vi "string parse mathematica list assosiated array.vi"(6 "pattern":string="[\\\\\\s\\n]*(\\d+)[\\\\\\s\\n]*\\-\\>[\\\\\\s\\n]*\\<\\|((.|\\n)+?)\\|\\>[\\\\\\s\\n]*\\,", 7 "derivative":T2=enum."parse string", 8 "array of inds":dbl[](array[numeric]), 10 "Map IN":map{i32, map{T1, dbl}}(c390), 11 "string IN":string="\n8048 -> <|\"\\[Zeta]\" -> 0.264284777894, \"\\[Tau]1\" -> 0.029921918685, \n   \"\\[Tau]S\" -> 0.192386764745, \"\\[Tau]N\" -> 0.181403587913, \n   \"\\[Tau]C\" -> 0.001052808010, \"\\[Kappa]0\" -> 0.000000000660, \n   \"mm1\" -> 0.000000000000, \"mm2\" -> 0.000000000000, \n   \"mm3\" -> 0.000000000000, \"T\" -> 0.170000000000, \n   \"B\" -> 12, \"\\[Theta]\" -> 0.000000000000|>, \n8049 -> <|\"\\[Zeta]\" -> 0.201102232421, \"\\[Tau]1\" -> 0.027404257658, \n   \"\\[Tau]S\" -> 0.119081991530, \"\\[Tau]N\" -> 0.102233037825, \n   \"\\[Tau]C\" -> 0.001034759526, \"\\[Kappa]0\" -> 0.000000000924, \n   \"mm1\" -> 0.000000000000, \"mm2\" -> 0.000000000000, \n   \"mm3\" -> 0.000000000000, \"T\" -> 0.200000000000, \n   \"B\" -> 12, \"\\[Theta]\" -> 0.000000000000|>, \n8050 -> <|\"\\[Zeta]\" -> 0.169063131197, \"\\[Tau]1\" -> 0.023551252455, \n   \"\\[Tau]S\" -> 0.088556796938, \"\\[Tau]N\" -> 0.073591360902, \n   \"\\[Tau]C\" -> 0.001008773464, \"\\[Kappa]0\" -> 0.000000001052, \n   \"mm1\" -> 0.000000000000, \"mm2\" -> 0.000000000000, \n   \"mm3\" -> 0.000000000000, \"T\" -> 0.220000000000, \n   \"B\" -> 12, \"\\[Theta]\" -> 0.000000000000|>, \n8051 -> <|\"\\[Zeta]\" -> 0.091539753140, \"\\[Tau]1\" -> 0.021589342173, \n   \"\\[Tau]S\" -> 0.069591266812, \"\\[Tau]N\" -> 0.024713101747, \n   \"\\[Tau]C\" -> 0.001578835918, \"\\[Kappa]0\" -> 0.000000001376, \n   \"mm1\" -> 0.000000000000, \"mm2\" -> 0.000000000000, \n   \"mm3\" -> 0.000000000000, \"T\" -> 0.280000000000, \n   \"B\" -> 12, \"\\[Theta]\" -> 0.000000000000|>, \n8052 -> <|\"\\[Zeta]\" -> 0.064241434685, \"\\[Tau]1\" -> 0.021883189624, \n   \"\\[Tau]S\" -> 0.054526069267, \"\\[Tau]N\" -> 0.012051949674, \n   \"\\[Tau]C\" -> 0.001858120134, \"\\[Kappa]0\" -> 0.000000001749, \n   \"mm1\" -> 0.000000000000, \"mm2\" -> 0.000000000000, \n   \"mm3\" -> 0.000000000000, \"T\" -> 0.330000000000, \n   \"B\" -> 12, \"\\[Theta]\" -> 0.000000000000|>, \n8053 -> <|\"\\[Zeta]\" -> 0.046671238462, \"\\[Tau]1\" -> 0.021035137247, \n   \"\\[Tau]S\" -> 0.044251032051, \"\\[Tau]N\" -> 0.006393660877, \n   \"\\[Tau]C\" -> 0.002341606240, \"\\[Kappa]0\" -> 0.000000002165, \n   \"mm1\" -> 0.000000000000, \"mm2\" -> 0.000000000000, \n   \"mm3\" -> 0.000000000000, \"T\" -> 0.400000000000, \n   \"B\" -> 12, \"\\[Theta]\" -> 0.000000000000|>, \n 8054 -> <|\"\\[Zeta]\" -> 0.036507468942, \"\\[Tau]1\" -> 0.016809078537, \n   \"\\[Tau]S\" -> 0.036180977899, \"\\[Tau]N\" -> 0.004191377428, \n   \"\\[Tau]C\" -> 0.002304673955, \"\\[Kappa]0\" -> 0.000000002675, \n   \"mm1\" -> 0.000000000000, \"mm2\" -> 0.000000000000, \n   \"mm3\" -> 0.000000000000, \"T\" -> 0.480000000000, \n   \"B\" -> 12, \"\\[Theta]\" -> 0.000000000000|>, \n 8055 -> <|\"\\[Zeta]\" -> 0.030833243094, \"\\[Tau]1\" -> 0.018820733306, \n   \"\\[Tau]S\" -> 0.030309186701, \"\\[Tau]N\" -> 0.002241639015, \n   \"\\[Tau]C\" -> 0.002272740822, \"\\[Kappa]0\" -> 0.000000003352, \n   \"mm1\" -> 0.000000000000, \"mm2\" -> 0.000000000000, \n   \"mm3\" -> 0.000000000000, \"T\" -> 0.580000000000, \n   \"B\" -> 12, \"\\[Theta]\" -> 0.000000000000|>, \n 8056 -> <|\"\\[Zeta]\" -> 0.019920170845, \"\\[Tau]1\" -> 0.016368892412, \n   \"\\[Tau]S\" -> 0.030579536580, \"\\[Tau]N\" -> 0.001736017565, \n   \"\\[Tau]C\" -> 0.004971418152, \"\\[Kappa]0\" -> 0.000000004410, \n   \"mm1\" -> 0.000000000000, \"mm2\" -> 0.000000000000, \n   \"mm3\" -> 0.000000000000, \"T\" -> 0.680000000000, \n   \"B\" -> 12, \"\\[Theta]\" -> 0.000000000000|>, \n 8057 -> <|\"\\[Zeta]\" -> 0.017558473054, \"\\[Tau]1\" -> 0.014545104284, \n   \"\\[Tau]S\" -> 0.022979681288, \"\\[Tau]N\" -> 0.000840829385, \n   \"\\[Tau]C\" -> 0.005228030240, \"\\[Kappa]0\" -> 0.000000006068, \n   \"mm1\" -> 0.000000000000, \"mm2\" -> 0.000000000000, \n   \"mm3\" -> 0.000000000000, \"T\" -> 0.910000000000, \n   \"B\" -> 12, \"\\[Theta]\" -> 0.000000000000|>, \n 8058 -> <|\"\\[Zeta]\" -> 0.011916480594, \"\\[Tau]1\" -> 0.012551282481, \n   \"\\[Tau]S\" -> 0.018233218660, \"\\[Tau]N\" -> 0.000345702746, \n   \"\\[Tau]C\" -> 0.004699451527, \"\\[Kappa]0\" -> 0.000000008451, \n   \"mm1\" -> 0.000000000000, \"mm2\" -> 0.000000000000, \n   \"mm3\" -> 0.000000000000, \"T\" -> 1.230000000000, \n   \"B\" -> 12, \"\\[Theta]\" -> 0.000000000000|>, \n 8059 -> <|\"\\[Zeta]\" -> 0.012831327568, \"\\[Tau]1\" -> 0.013315909415, \n   \"\\[Tau]S\" -> 0.012590836847, \"\\[Tau]N\" -> 0.000065003013, \n   \"\\[Tau]C\" -> 0.005276356243, \"\\[Kappa]0\" -> 0.000000013610, \n   \"mm1\" -> 0.000000000000, \"mm2\" -> 0.000000000000, \n   \"mm3\" -> 0.000000000000, \"T\" -> 1.970000000000, \n   \"B\" -> 12, \"\\[Theta]\" -> 0.000000000000|>, \n 8060 -> <|\"\\[Zeta]\" -> 0.019774146838, \"\\[Tau]1\" -> 0.013257273421, \n   \"\\[Tau]S\" -> 0.007064131508, \"\\[Tau]N\" -> 0.000028000819, \n   \"\\[Tau]C\" -> 0.006942241845, \"\\[Kappa]0\" -> 0.000000023477, \n   \"mm1\" -> 0.000000000000, \"mm2\" -> 0.000000000000, \n   \"mm3\" -> 0.000000000000, \"T\" -> 3.190000000000, \n   \"B\" -> 12, \"\\[Theta]\" -> 0.000000000000|>, \n 8061 -> <|\"\\[Zeta]\" -> 0.029251354442, \"\\[Tau]1\" -> 0.014634751206, \n   \"\\[Tau]S\" -> 0.003873958746, \"\\[Tau]N\" -> 0.000007000487, \n   \"\\[Tau]C\" -> 0.006827504775, \"\\[Kappa]0\" -> 0.000000056438, \n   \"mm1\" -> 0.000000000000, \"mm2\" -> 0.000000000000, \n   \"mm3\" -> 0.000000000000, \"T\" -> 5.820000000000, \n   \"B\" -> 12, \"\\[Theta]\" -> 0.000000000000 |>, \n   \n 8070 -> <|\"\\[Zeta]\" -> 0.192260325342, \"\\[Tau]1\" -> 0.068971960572, \n   \"\\[Tau]S\" -> 0.034724103146, \"\\[Tau]N\" -> 0.116916926394, \n   \"\\[Tau]C\" -> 0.001339007531, \"\\[Kappa]0\" -> 0.000000000920, \n   \"mm1\" -> 0.000000000000, \"mm2\" -> 0.000000000000, \n   \"mm3\" -> 0.000000000000, \"T\" -> 0.200000000000, \n   \"B\" -> 12, \"\\[Theta]\" -> 90.000000000000 |>, \n   \n 8071 -> <|\"\\[Zeta]\" -> 0.287121975239, \"\\[Tau]1\" -> 0.116231019165, \n   \"\\[Tau]S\" -> 0.066964365948, \"\\[Tau]N\" -> 1.031943818405, \n   \"\\[Tau]C\" -> 0.001579683432, \"\\[Kappa]0\" -> 0.000000000546, \n   \"mm1\" -> 0.000000000000, \"mm2\" -> 0.000000000000, \n   \"mm3\" -> 0.000000000000, \"T\" -> 0.140000000000, \n   \"B\" -> 12, \"\\[Theta]\" -> 90.000000000000 |>, \n   \n 8072 -> <|\"\\[Zeta]\" -> 0.256563977847, \"\\[Tau]1\" -> 0.091128230148, \n   \"\\[Tau]S\" -> 0.042349271948, \"\\[Tau]N\" -> 0.264223732455, \n   \"\\[Tau]C\" -> 0.001175524600, \"\\[Kappa]0\" -> 0.000000000659, \n   \"mm1\" -> 0.000000000000, \"mm2\" -> 0.000000000000, \n   \"mm3\" -> 0.000000000000, \"T\" -> 0.180000000000, \n   \"B\" -> 12, \"\\[Theta]\" -> 90.000000000000|>, \n 8073 -> <|\"\\[Zeta]\" -> 0.166463706425, \"\\[Tau]1\" -> 0.068258677765, \n   \"\\[Tau]S\" -> 0.032169678694, \"\\[Tau]N\" -> 0.089325850968, \n   \"\\[Tau]C\" -> 0.001296501731, \"\\[Kappa]0\" -> 0.000000001072, \n   \"mm1\" -> 0.000000000000, \"mm2\" -> 0.000000000000, \n   \"mm3\" -> 0.000000000000, \"T\" -> 0.220000000000, \n   \"B\" -> 12, \"\\[Theta]\" -> 90.000000000000|>, \n 8074 -> <|\"\\[Zeta]\" -> 0.096966986681, \"\\[Tau]1\" -> 0.051268159149, \n   \"\\[Tau]S\" -> 0.027100433808, \"\\[Tau]N\" -> 0.035158364681, \n   \"\\[Tau]C\" -> 0.001794012368, \"\\[Kappa]0\" -> 0.000000001377, \n   \"mm1\" -> 0.000000000000, \"mm2\" -> 0.000000000000, \n   \"mm3\" -> 0.000000000000, \"T\" -> 0.270000000000, \n   \"B\" -> 12, \"\\[Theta]\" -> 90.000000000000|>, \n 8075 -> <|\"\\[Zeta]\" -> 0.069751073871, \"\\[Tau]1\" -> 0.043839592936, \n   \"\\[Tau]S\" -> 0.023745040482, \"\\[Tau]N\" -> 0.017573258627, \n   \"\\[Tau]C\" -> 0.001911807541, \"\\[Kappa]0\" -> 0.000000001743, \n   \"mm1\" -> 0.000000000000, \"mm2\" -> 0.000000000000, \n   \"mm3\" -> 0.000000000000, \"T\" -> 0.330000000000, \n   \"B\" -> 12, \"\\[Theta]\" -> 90.000000000000|>, \n 8076 -> <|\"\\[Zeta]\" -> 0.051456166730, \"\\[Tau]1\" -> 0.036962114127, \n   \"\\[Tau]S\" -> 0.021589166615, \"\\[Tau]N\" -> 0.010172333923, \n   \"\\[Tau]C\" -> 0.002367575609, \"\\[Kappa]0\" -> 0.000000002122, \n   \"mm1\" -> 0.000000000000, \"mm2\" -> 0.000000000000, \n   \"mm3\" -> 0.000000000000, \"T\" -> 0.390000000000, \n   \"B\" -> 12, \"\\[Theta]\" -> 90.000000000000|>, \n 8077 -> <|\"\\[Zeta]\" -> 0.038526442831, \"\\[Tau]1\" -> 0.026952038906, \n   \"\\[Tau]S\" -> 0.019853633024, \"\\[Tau]N\" -> 0.005229312619, \n   \"\\[Tau]C\" -> 0.002387050238, \"\\[Kappa]0\" -> 0.000000002669, \n   \"mm1\" -> 0.000000000000, \"mm2\" -> 0.000000000000, \n   \"mm3\" -> 0.000000000000, \"T\" -> 0.480000000000, \n   \"B\" -> 12, \"\\[Theta]\" -> 90.000000000000|>, \n 8078 -> <|\"\\[Zeta]\" -> 0.031217986851, \"\\[Tau]1\" -> 0.022324330444, \n   \"\\[Tau]S\" -> 0.018861062526, \"\\[Tau]N\" -> 0.002718571339, \n   \"\\[Tau]C\" -> 0.002455004531, \"\\[Kappa]0\" -> 0.000000003343, \n   \"mm1\" -> 0.000000000000, \"mm2\" -> 0.000000000000, \n   \"mm3\" -> 0.000000000000, \"T\" -> 0.580000000000, \n   \"B\" -> 12, \"\\[Theta]\" -> 90.000000000000|>, \n 8079 -> <|\"\\[Zeta]\" -> 0.020568815513, \"\\[Tau]1\" -> 0.023045965648, \n   \"\\[Tau]S\" -> 0.020791387386, \"\\[Tau]N\" -> 0.002229171297, \n   \"\\[Tau]C\" -> 0.004427475438, \"\\[Kappa]0\" -> 0.000000004398, \n   \"mm1\" -> 0.000000000000, \"mm2\" -> 0.000000000000, \n   \"mm3\" -> 0.000000000000, \"T\" -> 0.680000000000, \n   \"B\" -> 12, \"\\[Theta]\" -> 90.000000000000|>, \n 8080 -> <|\"\\[Zeta]\" -> 0.016159836955, \"\\[Tau]1\" -> 0.019958638777, \n   \"\\[Tau]S\" -> 0.018730096307, \"\\[Tau]N\" -> 0.000899236968, \n   \"\\[Tau]C\" -> 0.005152267403, \"\\[Kappa]0\" -> 0.000000006087, \n   \"mm1\" -> 0.000000000000, \"mm2\" -> 0.000000000000, \n   \"mm3\" -> 0.000000000000, \"T\" -> 0.910000000000, \n   \"B\" -> 12, \"\\[Theta]\" -> 90.000000000000|>, \n 8081 -> <|\"\\[Zeta]\" -> 0.014495870556, \"\\[Tau]1\" -> 0.019990087457, \n   \"\\[Tau]S\" -> 0.016832201384, \"\\[Tau]N\" -> 0.000455517238, \n   \"\\[Tau]C\" -> 0.005555782498, \"\\[Kappa]0\" -> 0.000000008420, \n   \"mm1\" -> 0.000000000000, \"mm2\" -> 0.000000000000, \n   \"mm3\" -> 0.000000000000, \"T\" -> 1.230000000000, \n   \"B\" -> 12, \"\\[Theta]\" -> 90.000000000000|>, \n 8082 -> <|\"\\[Zeta]\" -> 0.014043763709, \"\\[Tau]1\" -> 0.018292068543, \n   \"\\[Tau]S\" -> 0.011311396743, \"\\[Tau]N\" -> 0.000128802259, \n   \"\\[Tau]C\" -> 0.008087849636, \"\\[Kappa]0\" -> 0.000000014258, \n   \"mm1\" -> 0.000000000000, \"mm2\" -> 0.000000000000, \n   \"mm3\" -> 0.000000000000, \"T\" -> 2.050000000000, \n   \"B\" -> 12, \"\\[Theta]\" -> 90.000000000000|>, \n 8083 -> <|\"\\[Zeta]\" -> 0.016187684631, \"\\[Tau]1\" -> 0.018325345271, \n   \"\\[Tau]S\" -> 0.007510087776, \"\\[Tau]N\" -> 0.000028419157, \n   \"\\[Tau]C\" -> 0.008115463080, \"\\[Kappa]0\" -> 0.000000024747, \n   \"mm1\" -> 0.000000000000, \"mm2\" -> 0.000000000000, \n   \"mm3\" -> 0.000000000000, \"T\" -> 3.310000000000, \n   \"B\" -> 12, \"\\[Theta]\" -> 90.000000000000|>, \n 8084 -> <|\"\\[Zeta]\" -> 0.027897403691, \"\\[Tau]1\" -> 0.014639690770, \n   \"\\[Tau]S\" -> 0.004105291179, \"\\[Tau]N\" -> 0.000006999171, \n   \"\\[Tau]C\" -> 0.007414449545, \"\\[Kappa]0\" -> 0.000000059701, \n   \"mm1\" -> 0.000000000000, \"mm2\" -> 0.000000000000, \n   \"mm3\" -> 0.000000000000, \"T\" -> 6.000000000000, \n   \"B\" -> 12, \"\\[Theta]\" -> 90.000000000000|>,") -> (2 "Map OUT":map{i32, map{T1, dbl}}(c390), 3 "string out":string="\n8048 -> <|\"\\[Zeta]\" -> 0.264284777894, \"\\[Tau]1\" -> 0.029921918685, \n   \"\\[Tau]S\" -> 0.192386764745, \"\\[Tau]N\" -> 0.181403587913, \n   \"\\[Tau]C\" -> 0.001052808010, \"\\[Kappa]0\" -> 0.000000000660, \n   \"mm1\" -> 0.000000000000, \"mm2\" -> 0.000000000000, \n   \"mm3\" -> 0.000000000000, \"T\" -> 0.170000000000, \n   \"B\" -> 12, \"\\[Theta]\" -> 0.000000000000|>, \n8049 -> <|\"\\[Zeta]\" -> 0.201102232421, \"\\[Tau]1\" -> 0.027404257658, \n   \"\\[Tau]S\" -> 0.119081991530, \"\\[Tau]N\" -> 0.102233037825, \n   \"\\[Tau]C\" -> 0.001034759526, \"\\[Kappa]0\" -> 0.000000000924, \n   \"mm1\" -> 0.000000000000, \"mm2\" -> 0.000000000000, \n   \"mm3\" -> 0.000000000000, \"T\" -> 0.200000000000, \n   \"B\" -> 12, \"\\[Theta]\" -> 0.000000000000|>, \n8050 -> <|\"\\[Zeta]\" -> 0.169063131197, \"\\[Tau]1\" -> 0.023551252455, \n   \"\\[Tau]S\" -> 0.088556796938, \"\\[Tau]N\" -> 0.073591360902, \n   \"\\[Tau]C\" -> 0.001008773464, \"\\[Kappa]0\" -> 0.000000001052, \n   \"mm1\" -> 0.000000000000, \"mm2\" -> 0.000000000000, \n   \"mm3\" -> 0.000000000000, \"T\" -> 0.220000000000, \n   \"B\" -> 12, \"\\[Theta]\" -> 0.000000000000|>, \n8051 -> <|\"\\[Zeta]\" -> 0.091539753140, \"\\[Tau]1\" -> 0.021589342173, \n   \"\\[Tau]S\" -> 0.069591266812, \"\\[Tau]N\" -> 0.024713101747, \n   \"\\[Tau]C\" -> 0.001578835918, \"\\[Kappa]0\" -> 0.000000001376, \n   \"mm1\" -> 0.000000000000, \"mm2\" -> 0.000000000000, \n   \"mm3\" -> 0.000000000000, \"T\" -> 0.280000000000, \n   \"B\" -> 12, \"\\[Theta]\" -> 0.000000000000|>, \n8052 -> <|\"\\[Zeta]\" -> 0.064241434685, \"\\[Tau]1\" -> 0.021883189624, \n   \"\\[Tau]S\" -> 0.054526069267, \"\\[Tau]N\" -> 0.012051949674, \n   \"\\[Tau]C\" -> 0.001858120134, \"\\[Kappa]0\" -> 0.000000001749, \n   \"mm1\" -> 0.000000000000, \"mm2\" -> 0.000000000000, \n   \"mm3\" -> 0.000000000000, \"T\" -> 0.330000000000, \n   \"B\" -> 12, \"\\[Theta]\" -> 0.000000000000|>, \n8053 -> <|\"\\[Zeta]\" -> 0.046671238462, \"\\[Tau]1\" -> 0.021035137247, \n   \"\\[Tau]S\" -> 0.044251032051, \"\\[Tau]N\" -> 0.006393660877, \n   \"\\[Tau]C\" -> 0.002341606240, \"\\[Kappa]0\" -> 0.000000002165, \n   \"mm1\" -> 0.000000000000, \"mm2\" -> 0.000000000000, \n   \"mm3\" -> 0.000000000000, \"T\" -> 0.400000000000, \n   \"B\" -> 12, \"\\[Theta]\" -> 0.000000000000|>, \n 8054 -> <|\"\\[Zeta]\" -> 0.036507468942, \"\\[Tau]1\" -> 0.016809078537, \n   \"\\[Tau]S\" -> 0.036180977899, \"\\[Tau]N\" -> 0.004191377428, \n   \"\\[Tau]C\" -> 0.002304673955, \"\\[Kappa]0\" -> 0.000000002675, \n   \"mm1\" -> 0.000000000000, \"mm2\" -> 0.000000000000, \n   \"mm3\" -> 0.000000000000, \"T\" -> 0.480000000000, \n   \"B\" -> 12, \"\\[Theta]\" -> 0.000000000000|>, \n 8055 -> <|\"\\[Zeta]\" -> 0.030833243094, \"\\[Tau]1\" -> 0.018820733306, \n   \"\\[Tau]S\" -> 0.030309186701, \"\\[Tau]N\" -> 0.002241639015, \n   \"\\[Tau]C\" -> 0.002272740822, \"\\[Kappa]0\" -> 0.000000003352, \n   \"mm1\" -> 0.000000000000, \"mm2\" -> 0.000000000000, \n   \"mm3\" -> 0.000000000000, \"T\" -> 0.580000000000, \n   \"B\" -> 12, \"\\[Theta]\" -> 0.000000000000|>, \n 8056 -> <|\"\\[Zeta]\" -> 0.019920170845, \"\\[Tau]1\" -> 0.016368892412, \n   \"\\[Tau]S\" -> 0.030579536580, \"\\[Tau]N\" -> 0.001736017565, \n   \"\\[Tau]C\" -> 0.004971418152, \"\\[Kappa]0\" -> 0.000000004410, \n   \"mm1\" -> 0.000000000000, \"mm2\" -> 0.000000000000, \n   \"mm3\" -> 0.000000000000, \"T\" -> 0.680000000000, \n   \"B\" -> 12, \"\\[Theta]\" -> 0.000000000000|>, \n 8057 -> <|\"\\[Zeta]\" -> 0.017558473054, \"\\[Tau]1\" -> 0.014545104284, \n   \"\\[Tau]S\" -> 0.022979681288, \"\\[Tau]N\" -> 0.000840829385, \n   \"\\[Tau]C\" -> 0.005228030240, \"\\[Kappa]0\" -> 0.000000006068, \n   \"mm1\" -> 0.000000000000, \"mm2\" -> 0.000000000000, \n   \"mm3\" -> 0.000000000000, \"T\" -> 0.910000000000, \n   \"B\" -> 12, \"\\[Theta]\" -> 0.000000000000|>, \n 8058 -> <|\"\\[Zeta]\" -> 0.011916480594, \"\\[Tau]1\" -> 0.012551282481, \n   \"\\[Tau]S\" -> 0.018233218660, \"\\[Tau]N\" -> 0.000345702746, \n   \"\\[Tau]C\" -> 0.004699451527, \"\\[Kappa]0\" -> 0.000000008451, \n   \"mm1\" -> 0.000000000000, \"mm2\" -> 0.000000000000, \n   \"mm3\" -> 0.000000000000, \"T\" -> 1.230000000000, \n   \"B\" -> 12, \"\\[Theta]\" -> 0.000000000000|>, \n 8059 -> <|\"\\[Zeta]\" -> 0.012831327568, \"\\[Tau]1\" -> 0.013315909415, \n   \"\\[Tau]S\" -> 0.012590836847, \"\\[Tau]N\" -> 0.000065003013, \n   \"\\[Tau]C\" -> 0.005276356243, \"\\[Kappa]0\" -> 0.000000013610, \n   \"mm1\" -> 0.000000000000, \"mm2\" -> 0.000000000000, \n   \"mm3\" -> 0.000000000000, \"T\" -> 1.970000000000, \n   \"B\" -> 12, \"\\[Theta]\" -> 0.000000000000|>, \n 8060 -> <|\"\\[Zeta]\" -> 0.019774146838, \"\\[Tau]1\" -> 0.013257273421, \n   \"\\[Tau]S\" -> 0.007064131508, \"\\[Tau]N\" -> 0.000028000819, \n   \"\\[Tau]C\" -> 0.006942241845, \"\\[Kappa]0\" -> 0.000000023477, \n   \"mm1\" -> 0.000000000000, \"mm2\" -> 0.000000000000, \n   \"mm3\" -> 0.000000000000, \"T\" -> 3.190000000000, \n   \"B\" -> 12, \"\\[Theta]\" -> 0.000000000000|>, \n 8061 -> <|\"\\[Zeta]\" -> 0.029251354442, \"\\[Tau]1\" -> 0.014634751206, \n   \"\\[Tau]S\" -> 0.003873958746, \"\\[Tau]N\" -> 0.000007000487, \n   \"\\[Tau]C\" -> 0.006827504775, \"\\[Kappa]0\" -> 0.000000056438, \n   \"mm1\" -> 0.000000000000, \"mm2\" -> 0.000000000000, \n   \"mm3\" -> 0.000000000000, \"T\" -> 5.820000000000, \n   \"B\" -> 12, \"\\[Theta]\" -> 0.000000000000 |>, \n   \n 8070 -> <|\"\\[Zeta]\" -> 0.192260325342, \"\\[Tau]1\" -> 0.068971960572, \n   \"\\[Tau]S\" -> 0.034724103146, \"\\[Tau]N\" -> 0.116916926394, \n   \"\\[Tau]C\" -> 0.001339007531, \"\\[Kappa]0\" -> 0.000000000920, \n   \"mm1\" -> 0.000000000000, \"mm2\" -> 0.000000000000, \n   \"mm3\" -> 0.000000000000, \"T\" -> 0.200000000000, \n   \"B\" -> 12, \"\\[Theta]\" -> 90.000000000000 |>, \n   \n 8071 -> <|\"\\[Zeta]\" -> 0.287121975239, \"\\[Tau]1\" -> 0.116231019165, \n   \"\\[Tau]S\" -> 0.066964365948, \"\\[Tau]N\" -> 1.031943818405, \n   \"\\[Tau]C\" -> 0.001579683432, \"\\[Kappa]0\" -> 0.000000000546, \n   \"mm1\" -> 0.000000000000, \"mm2\" -> 0.000000000000, \n   \"mm3\" -> 0.000000000000, \"T\" -> 0.140000000000, \n   \"B\" -> 12, \"\\[Theta]\" -> 90.000000000000 |>, \n   \n 8072 -> <|\"\\[Zeta]\" -> 0.256563977847, \"\\[Tau]1\" -> 0.091128230148, \n   \"\\[Tau]S\" -> 0.042349271948, \"\\[Tau]N\" -> 0.264223732455, \n   \"\\[Tau]C\" -> 0.001175524600, \"\\[Kappa]0\" -> 0.000000000659, \n   \"mm1\" -> 0.000000000000, \"mm2\" -> 0.000000000000, \n   \"mm3\" -> 0.000000000000, \"T\" -> 0.180000000000, \n   \"B\" -> 12, \"\\[Theta]\" -> 90.000000000000|>, \n 8073 -> <|\"\\[Zeta]\" -> 0.166463706425, \"\\[Tau]1\" -> 0.068258677765, \n   \"\\[Tau]S\" -> 0.032169678694, \"\\[Tau]N\" -> 0.089325850968, \n   \"\\[Tau]C\" -> 0.001296501731, \"\\[Kappa]0\" -> 0.000000001072, \n   \"mm1\" -> 0.000000000000, \"mm2\" -> 0.000000000000, \n   \"mm3\" -> 0.000000000000, \"T\" -> 0.220000000000, \n   \"B\" -> 12, \"\\[Theta]\" -> 90.000000000000|>, \n 8074 -> <|\"\\[Zeta]\" -> 0.096966986681, \"\\[Tau]1\" -> 0.051268159149, \n   \"\\[Tau]S\" -> 0.027100433808, \"\\[Tau]N\" -> 0.035158364681, \n   \"\\[Tau]C\" -> 0.001794012368, \"\\[Kappa]0\" -> 0.000000001377, \n   \"mm1\" -> 0.000000000000, \"mm2\" -> 0.000000000000, \n   \"mm3\" -> 0.000000000000, \"T\" -> 0.270000000000, \n   \"B\" -> 12, \"\\[Theta]\" -> 90.000000000000|>, \n 8075 -> <|\"\\[Zeta]\" -> 0.069751073871, \"\\[Tau]1\" -> 0.043839592936, \n   \"\\[Tau]S\" -> 0.023745040482, \"\\[Tau]N\" -> 0.017573258627, \n   \"\\[Tau]C\" -> 0.001911807541, \"\\[Kappa]0\" -> 0.000000001743, \n   \"mm1\" -> 0.000000000000, \"mm2\" -> 0.000000000000, \n   \"mm3\" -> 0.000000000000, \"T\" -> 0.330000000000, \n   \"B\" -> 12, \"\\[Theta]\" -> 90.000000000000|>, \n 8076 -> <|\"\\[Zeta]\" -> 0.051456166730, \"\\[Tau]1\" -> 0.036962114127, \n   \"\\[Tau]S\" -> 0.021589166615, \"\\[Tau]N\" -> 0.010172333923, \n   \"\\[Tau]C\" -> 0.002367575609, \"\\[Kappa]0\" -> 0.000000002122, \n   \"mm1\" -> 0.000000000000, \"mm2\" -> 0.000000000000, \n   \"mm3\" -> 0.000000000000, \"T\" -> 0.390000000000, \n   \"B\" -> 12, \"\\[Theta]\" -> 90.000000000000|>, \n 8077 -> <|\"\\[Zeta]\" -> 0.038526442831, \"\\[Tau]1\" -> 0.026952038906, \n   \"\\[Tau]S\" -> 0.019853633024, \"\\[Tau]N\" -> 0.005229312619, \n   \"\\[Tau]C\" -> 0.002387050238, \"\\[Kappa]0\" -> 0.000000002669, \n   \"mm1\" -> 0.000000000000, \"mm2\" -> 0.000000000000, \n   \"mm3\" -> 0.000000000000, \"T\" -> 0.480000000000, \n   \"B\" -> 12, \"\\[Theta]\" -> 90.000000000000|>, \n 8078 -> <|\"\\[Zeta]\" -> 0.031217986851, \"\\[Tau]1\" -> 0.022324330444, \n   \"\\[Tau]S\" -> 0.018861062526, \"\\[Tau]N\" -> 0.002718571339, \n   \"\\[Tau]C\" -> 0.002455004531, \"\\[Kappa]0\" -> 0.000000003343, \n   \"mm1\" -> 0.000000000000, \"mm2\" -> 0.000000000000, \n   \"mm3\" -> 0.000000000000, \"T\" -> 0.580000000000, \n   \"B\" -> 12, \"\\[Theta]\" -> 90.000000000000|>, \n 8079 -> <|\"\\[Zeta]\" -> 0.020568815513, \"\\[Tau]1\" -> 0.023045965648, \n   \"\\[Tau]S\" -> 0.020791387386, \"\\[Tau]N\" -> 0.002229171297, \n   \"\\[Tau]C\" -> 0.004427475438, \"\\[Kappa]0\" -> 0.000000004398, \n   \"mm1\" -> 0.000000000000, \"mm2\" -> 0.000000000000, \n   \"mm3\" -> 0.000000000000, \"T\" -> 0.680000000000, \n   \"B\" -> 12, \"\\[Theta]\" -> 90.000000000000|>, \n 8080 -> <|\"\\[Zeta]\" -> 0.016159836955, \"\\[Tau]1\" -> 0.019958638777, \n   \"\\[Tau]S\" -> 0.018730096307, \"\\[Tau]N\" -> 0.000899236968, \n   \"\\[Tau]C\" -> 0.005152267403, \"\\[Kappa]0\" -> 0.000000006087, \n   \"mm1\" -> 0.000000000000, \"mm2\" -> 0.000000000000, \n   \"mm3\" -> 0.000000000000, \"T\" -> 0.910000000000, \n   \"B\" -> 12, \"\\[Theta]\" -> 90.000000000000|>, \n 8081 -> <|\"\\[Zeta]\" -> 0.014495870556, \"\\[Tau]1\" -> 0.019990087457, \n   \"\\[Tau]S\" -> 0.016832201384, \"\\[Tau]N\" -> 0.000455517238, \n   \"\\[Tau]C\" -> 0.005555782498, \"\\[Kappa]0\" -> 0.000000008420, \n   \"mm1\" -> 0.000000000000, \"mm2\" -> 0.000000000000, \n   \"mm3\" -> 0.000000000000, \"T\" -> 1.230000000000, \n   \"B\" -> 12, \"\\[Theta]\" -> 90.000000000000|>, \n 8082 -> <|\"\\[Zeta]\" -> 0.014043763709, \"\\[Tau]1\" -> 0.018292068543, \n   \"\\[Tau]S\" -> 0.011311396743, \"\\[Tau]N\" -> 0.000128802259, \n   \"\\[Tau]C\" -> 0.008087849636, \"\\[Kappa]0\" -> 0.000000014258, \n   \"mm1\" -> 0.000000000000, \"mm2\" -> 0.000000000000, \n   \"mm3\" -> 0.000000000000, \"T\" -> 2.050000000000, \n   \"B\" -> 12, \"\\[Theta]\" -> 90.000000000000|>, \n 8083 -> <|\"\\[Zeta]\" -> 0.016187684631, \"\\[Tau]1\" -> 0.018325345271, \n   \"\\[Tau]S\" -> 0.007510087776, \"\\[Tau]N\" -> 0.000028419157, \n   \"\\[Tau]C\" -> 0.008115463080, \"\\[Kappa]0\" -> 0.000000024747, \n   \"mm1\" -> 0.000000000000, \"mm2\" -> 0.000000000000, \n   \"mm3\" -> 0.000000000000, \"T\" -> 3.310000000000, \n   \"B\" -> 12, \"\\[Theta]\" -> 90.000000000000|>, \n 8084 -> <|\"\\[Zeta]\" -> 0.027897403691, \"\\[Tau]1\" -> 0.014639690770, \n   \"\\[Tau]S\" -> 0.004105291179, \"\\[Tau]N\" -> 0.000006999171, \n   \"\\[Tau]C\" -> 0.007414449545, \"\\[Kappa]0\" -> 0.000000059701, \n   \"mm1\" -> 0.000000000000, \"mm2\" -> 0.000000000000, \n   \"mm3\" -> 0.000000000000, \"T\" -> 6.000000000000, \n   \"B\" -> 12, \"\\[Theta]\" -> 90.000000000000|>,")   [LabVIEW 2020]
uses:
  3-lorentzian-parameters.ctl
  3-lorentzian-heat-response action.ctl
  mathematica string map action.ctl
  3-lorentzian-heat-response -- V4.vi/142dd4c5-f9ed-c64b-bc14-a88e3e2c450a.vi
  <vilib>/Analysis/polynomials.llb/Multiply Polynomials.vi
  <vilib>/Analysis/polynomials.llb/Multiply Polynomials (DBL).vi
  <vilib>/Analysis/polynomials.llb/Polynomial Roots.vi
  <vilib>/Analysis/polynomials.llb/Polynomial Roots (DBL).vi
  <vilib>/Comparison/Less/Less Functor/Less Functor.lvclass
  <vilib>/regexp/Match Regular Expression.xnode
panel:
  out "after match":string
  out "map of strings":map{i32, string}(c390)={8048="\"\\[Zeta]\" -> 0.264284777894, \"\\[Tau]1\" -> 0.029921918685, \n   \"\\[Tau]S\" -> 0.192386764745, \"\\[Tau]N\" -> 0.181403587913, \n   \"\\[Tau]C\" -> 0.001052808010, \"\\[Kappa]0\" -> 0.000000000660, \n   \"mm1\" -> 0.000000000000, \"mm2\" -> 0.000000000000, \n   \"mm3\" -> 0.000000000000, \"T\" -> 0.170000000000, \n   \"B\" -> 12, \"\\[Theta]\" -> 0.000000000000", 8049="\"\\[Zeta]\" -> 0.201102232421, \"\\[Tau]1\" -> 0.027404257658, \n   \"\\[Tau]S\" -> 0.119081991530, \"\\[Tau]N\" -> 0.102233037825, \n   \"\\[Tau]C\" -> 0.001034759526, \"\\[Kappa]0\" -> 0.000000000924, \n   \"mm1\" -> 0.000000000000, \"mm2\" -> 0.000000000000, \n   \"mm3\" -> 0.000000000000, \"T\" -> 0.200000000000, \n   \"B\" -> 12, \"\\[Theta]\" -> 0.000000000000", 8050="\"\\[Zeta]\" -> 0.169063131197, \"\\[Tau]1\" -> 0.023551252455, \n   \"\\[Tau]S\" -> 0.088556796938, \"\\[Tau]N\" -> 0.073591360902, \n   \"\\[Tau]C\" -> 0.001008773464, \"\\[Kappa]0\" -> 0.000000001052, \n   \"mm1\" -> 0.000000000000, \"mm2\" -> 0.000000000000, \n   \"mm3\" -> 0.000000000000, \"T\" -> 0.220000000000, \n   \"B\" -> 12, \"\\[Theta]\" -> 0.000000000000", 8051="\"\\[Zeta]\" -> 0.091539753140, \"\\[Tau]1\" -> 0.021589342173, \n   \"\\[Tau]S\" -> 0.069591266812, \"\\[Tau]N\" -> 0.024713101747, \n   \"\\[Tau]C\" -> 0.001578835918, \"\\[Kappa]0\" -> 0.000000001376, \n   \"mm1\" -> 0.000000000000, \"mm2\" -> 0.000000000000, \n   \"mm3\" -> 0.000000000000, \"T\" -> 0.280000000000, \n   \"B\" -> 12, \"\\[Theta]\" -> 0.000000000000", 8052="\"\\[Zeta]\" -> 0.064241434685, \"\\[Tau]1\" -> 0.021883189624, \n   \"\\[Tau]S\" -> 0.054526069267, \"\\[Tau]N\" -> 0.012051949674, \n   \"\\[Tau]C\" -> 0.001858120134, \"\\[Kappa]0\" -> 0.000000001749, \n   \"mm1\" -> 0.000000000000, \"mm2\" -> 0.000000000000, \n   \"mm3\" -> 0.000000000000, \"T\" -> 0.330000000000, \n   \"B\" -> 12, \"\\[Theta]\" -> 0.000000000000", 8053="\"\\[Zeta]\" -> 0.046671238462, \"\\[Tau]1\" -> 0.021035137247, \n   \"\\[Tau]S\" -> 0.044251032051, \"\\[Tau]N\" -> 0.006393660877, \n   \"\\[Tau]C\" -> 0.002341606240, \"\\[Kappa]0\" -> 0.000000002165, \n   \"mm1\" -> 0.000000000000, \"mm2\" -> 0.000000000000, \n   \"mm3\" -> 0.000000000000, \"T\" -> 0.400000000000, \n   \"B\" -> 12, \"\\[Theta]\" -> 0.000000000000", 8054="\"\\[Zeta]\" -> 0.036507468942, \"\\[Tau]1\" -> 0.016809078537, \n   \"\\[Tau]S\" -> 0.036180977899, \"\\[Tau]N\" -> 0.004191377428, \n   \"\\[Tau]C\" -> 0.002304673955, \"\\[Kappa]0\" -> 0.000000002675, \n   \"mm1\" -> 0.000000000000, \"mm2\" -> 0.000000000000, \n   \"mm3\" -> 0.000000000000, \"T\" -> 0.480000000000, \n   \"B\" -> 12, \"\\[Theta]\" -> 0.000000000000", 8055="\"\\[Zeta]\" -> 0.030833243094, \"\\[Tau]1\" -> 0.018820733306, \n   \"\\[Tau]S\" -> 0.030309186701, \"\\[Tau]N\" -> 0.002241639015, \n   \"\\[Tau]C\" -> 0.002272740822, \"\\[Kappa]0\" -> 0.000000003352, \n   \"mm1\" -> 0.000000000000, \"mm2\" -> 0.000000000000, \n   \"mm3\" -> 0.000000000000, \"T\" -> 0.580000000000, \n   \"B\" -> 12, \"\\[Theta]\" -> 0.000000000000", 8056="\"\\[Zeta]\" -> 0.019920170845, \"\\[Tau]1\" -> 0.016368892412, \n   \"\\[Tau]S\" -> 0.030579536580, \"\\[Tau]N\" -> 0.001736017565, \n   \"\\[Tau]C\" -> 0.004971418152, \"\\[Kappa]0\" -> 0.000000004410, \n   \"mm1\" -> 0.000000000000, \"mm2\" -> 0.000000000000, \n   \"mm3\" -> 0.000000000000, \"T\" -> 0.680000000000, \n   \"B\" -> 12, \"\\[Theta]\" -> 0.000000000000", 8057="\"\\[Zeta]\" -> 0.017558473054, \"\\[Tau]1\" -> 0.014545104284, \n   \"\\[Tau]S\" -> 0.022979681288, \"\\[Tau]N\" -> 0.000840829385, \n   \"\\[Tau]C\" -> 0.005228030240, \"\\[Kappa]0\" -> 0.000000006068, \n   \"mm1\" -> 0.000000000000, \"mm2\" -> 0.000000000000, \n   \"mm3\" -> 0.000000000000, \"T\" -> 0.910000000000, \n   \"B\" -> 12, \"\\[Theta]\" -> 0.000000000000", 8058="\"\\[Zeta]\" -> 0.011916480594, \"\\[Tau]1\" -> 0.012551282481, \n   \"\\[Tau]S\" -> 0.018233218660, \"\\[Tau]N\" -> 0.000345702746, \n   \"\\[Tau]C\" -> 0.004699451527, \"\\[Kappa]0\" -> 0.000000008451, \n   \"mm1\" -> 0.000000000000, \"mm2\" -> 0.000000000000, \n   \"mm3\" -> 0.000000000000, \"T\" -> 1.230000000000, \n   \"B\" -> 12, \"\\[Theta]\" -> 0.000000000000", 8059="\"\\[Zeta]\" -> 0.012831327568, \"\\[Tau]1\" -> 0.013315909415, \n   \"\\[Tau]S\" -> 0.012590836847, \"\\[Tau]N\" -> 0.000065003013, \n   \"\\[Tau]C\" -> 0.005276356243, \"\\[Kappa]0\" -> 0.000000013610, \n   \"mm1\" -> 0.000000000000, \"mm2\" -> 0.000000000000, \n   \"mm3\" -> 0.000000000000, \"T\" -> 1.970000000000, \n   \"B\" -> 12, \"\\[Theta]\" -> 0.000000000000", 8060="\"\\[Zeta]\" -> 0.019774146838, \"\\[Tau]1\" -> 0.013257273421, \n   \"\\[Tau]S\" -> 0.007064131508, \"\\[Tau]N\" -> 0.000028000819, \n   \"\\[Tau]C\" -> 0.006942241845, \"\\[Kappa]0\" -> 0.000000023477, \n   \"mm1\" -> 0.000000000000, \"mm2\" -> 0.000000000000, \n   \"mm3\" -> 0.000000000000, \"T\" -> 3.190000000000, \n   \"B\" -> 12, \"\\[Theta]\" -> 0.000000000000", 8061="\"\\[Zeta]\" -> 0.029251354442, \"\\[Tau]1\" -> 0.014634751206, \n   \"\\[Tau]S\" -> 0.003873958746, \"\\[Tau]N\" -> 0.000007000487, \n   \"\\[Tau]C\" -> 0.006827504775, \"\\[Kappa]0\" -> 0.000000056438, \n   \"mm1\" -> 0.000000000000, \"mm2\" -> 0.000000000000, \n   \"mm3\" -> 0.000000000000, \"T\" -> 5.820000000000, \n   \"B\" -> 12, \"\\[Theta]\" -> 0.000000000000 ", 8070="\"\\[Zeta]\" -> 0.192260325342, \"\\[Tau]1\" -> 0.068971960572, \n   \"\\[Tau]S\" -> 0.034724103146, \"\\[Tau]N\" -> 0.116916926394, \n   \"\\[Tau]C\" -> 0.001339007531, \"\\[Kappa]0\" -> 0.000000000920, \n   \"mm1\" -> 0.000000000000, \"mm2\" -> 0.000000000000, \n   \"mm3\" -> 0.000000000000, \"T\" -> 0.200000000000, \n   \"B\" -> 12, \"\\[Theta]\" -> 90.000000000000 ", 8071="\"\\[Zeta]\" -> 0.287121975239, \"\\[Tau]1\" -> 0.116231019165, \n   \"\\[Tau]S\" -> 0.066964365948, \"\\[Tau]N\" -> 1.031943818405, \n   \"\\[Tau]C\" -> 0.001579683432, \"\\[Kappa]0\" -> 0.000000000546, \n   \"mm1\" -> 0.000000000000, \"mm2\" -> 0.000000000000, \n   \"mm3\" -> 0.000000000000, \"T\" -> 0.140000000000, \n   \"B\" -> 12, \"\\[Theta]\" -> 90.000000000000 ", 8072="\"\\[Zeta]\" -> 0.256563977847, \"\\[Tau]1\" -> 0.091128230148, \n   \"\\[Tau]S\" -> 0.042349271948, \"\\[Tau]N\" -> 0.264223732455, \n   \"\\[Tau]C\" -> 0.001175524600, \"\\[Kappa]0\" -> 0.000000000659, \n   \"mm1\" -> 0.000000000000, \"mm2\" -> 0.000000000000, \n   \"mm3\" -> 0.000000000000, \"T\" -> 0.180000000000, \n   \"B\" -> 12, \"\\[Theta]\" -> 90.000000000000", 8073="\"\\[Zeta]\" -> 0.166463706425, \"\\[Tau]1\" -> 0.068258677765, \n   \"\\[Tau]S\" -> 0.032169678694, \"\\[Tau]N\" -> 0.089325850968, \n   \"\\[Tau]C\" -> 0.001296501731, \"\\[Kappa]0\" -> 0.000000001072, \n   \"mm1\" -> 0.000000000000, \"mm2\" -> 0.000000000000, \n   \"mm3\" -> 0.000000000000, \"T\" -> 0.220000000000, \n   \"B\" -> 12, \"\\[Theta]\" -> 90.000000000000", 8074="\"\\[Zeta]\" -> 0.096966986681, \"\\[Tau]1\" -> 0.051268159149, \n   \"\\[Tau]S\" -> 0.027100433808, \"\\[Tau]N\" -> 0.035158364681, \n   \"\\[Tau]C\" -> 0.001794012368, \"\\[Kappa]0\" -> 0.000000001377, \n   \"mm1\" -> 0.000000000000, \"mm2\" -> 0.000000000000, \n   \"mm3\" -> 0.000000000000, \"T\" -> 0.270000000000, \n   \"B\" -> 12, \"\\[Theta]\" -> 90.000000000000", 8075="\"\\[Zeta]\" -> 0.069751073871, \"\\[Tau]1\" -> 0.043839592936, \n   \"\\[Tau]S\" -> 0.023745040482, \"\\[Tau]N\" -> 0.017573258627, \n   \"\\[Tau]C\" -> 0.001911807541, \"\\[Kappa]0\" -> 0.000000001743, \n   \"mm1\" -> 0.000000000000, \"mm2\" -> 0.000000000000, \n   \"mm3\" -> 0.000000000000, \"T\" -> 0.330000000000, \n   \"B\" -> 12, \"\\[Theta]\" -> 90.000000000000", 8076="\"\\[Zeta]\" -> 0.051456166730, \"\\[Tau]1\" -> 0.036962114127, \n   \"\\[Tau]S\" -> 0.021589166615, \"\\[Tau]N\" -> 0.010172333923, \n   \"\\[Tau]C\" -> 0.002367575609, \"\\[Kappa]0\" -> 0.000000002122, \n   \"mm1\" -> 0.000000000000, \"mm2\" -> 0.000000000000, \n   \"mm3\" -> 0.000000000000, \"T\" -> 0.390000000000, \n   \"B\" -> 12, \"\\[Theta]\" -> 90.000000000000", 8077="\"\\[Zeta]\" -> 0.038526442831, \"\\[Tau]1\" -> 0.026952038906, \n   \"\\[Tau]S\" -> 0.019853633024, \"\\[Tau]N\" -> 0.005229312619, \n   \"\\[Tau]C\" -> 0.002387050238, \"\\[Kappa]0\" -> 0.000000002669, \n   \"mm1\" -> 0.000000000000, \"mm2\" -> 0.000000000000, \n   \"mm3\" -> 0.000000000000, \"T\" -> 0.480000000000, \n   \"B\" -> 12, \"\\[Theta]\" -> 90.000000000000", 8078="\"\\[Zeta]\" -> 0.031217986851, \"\\[Tau]1\" -> 0.022324330444, \n   \"\\[Tau]S\" -> 0.018861062526, \"\\[Tau]N\" -> 0.002718571339, \n   \"\\[Tau]C\" -> 0.002455004531, \"\\[Kappa]0\" -> 0.000000003343, \n   \"mm1\" -> 0.000000000000, \"mm2\" -> 0.000000000000, \n   \"mm3\" -> 0.000000000000, \"T\" -> 0.580000000000, \n   \"B\" -> 12, \"\\[Theta]\" -> 90.000000000000", 8079="\"\\[Zeta]\" -> 0.020568815513, \"\\[Tau]1\" -> 0.023045965648, \n   \"\\[Tau]S\" -> 0.020791387386, \"\\[Tau]N\" -> 0.002229171297, \n   \"\\[Tau]C\" -> 0.004427475438, \"\\[Kappa]0\" -> 0.000000004398, \n   \"mm1\" -> 0.000000000000, \"mm2\" -> 0.000000000000, \n   \"mm3\" -> 0.000000000000, \"T\" -> 0.680000000000, \n   \"B\" -> 12, \"\\[Theta]\" -> 90.000000000000", 8080="\"\\[Zeta]\" -> 0.016159836955, \"\\[Tau]1\" -> 0.019958638777, \n   \"\\[Tau]S\" -> 0.018730096307, \"\\[Tau]N\" -> 0.000899236968, \n   \"\\[Tau]C\" -> 0.005152267403, \"\\[Kappa]0\" -> 0.000000006087, \n   \"mm1\" -> 0.000000000000, \"mm2\" -> 0.000000000000, \n   \"mm3\" -> 0.000000000000, \"T\" -> 0.910000000000, \n   \"B\" -> 12, \"\\[Theta]\" -> 90.000000000000", 8081="\"\\[Zeta]\" -> 0.014495870556, \"\\[Tau]1\" -> 0.019990087457, \n   \"\\[Tau]S\" -> 0.016832201384, \"\\[Tau]N\" -> 0.000455517238, \n   \"\\[Tau]C\" -> 0.005555782498, \"\\[Kappa]0\" -> 0.000000008420, \n   \"mm1\" -> 0.000000000000, \"mm2\" -> 0.000000000000, \n   \"mm3\" -> 0.000000000000, \"T\" -> 1.230000000000, \n   \"B\" -> 12, \"\\[Theta]\" -> 90.000000000000", 8082="\"\\[Zeta]\" -> 0.014043763709, \"\\[Tau]1\" -> 0.018292068543, \n   \"\\[Tau]S\" -> 0.011311396743, \"\\[Tau]N\" -> 0.000128802259, \n   \"\\[Tau]C\" -> 0.008087849636, \"\\[Kappa]0\" -> 0.000000014258, \n   \"mm1\" -> 0.000000000000, \"mm2\" -> 0.000000000000, \n   \"mm3\" -> 0.000000000000, \"T\" -> 2.050000000000, \n   \"B\" -> 12, \"\\[Theta]\" -> 90.000000000000", 8083="\"\\[Zeta]\" -> 0.016187684631, \"\\[Tau]1\" -> 0.018325345271, \n   \"\\[Tau]S\" -> 0.007510087776, \"\\[Tau]N\" -> 0.000028419157, \n   \"\\[Tau]C\" -> 0.008115463080, \"\\[Kappa]0\" -> 0.000000024747, \n   \"mm1\" -> 0.000000000000, \"mm2\" -> 0.000000000000, \n   \"mm3\" -> 0.000000000000, \"T\" -> 3.310000000000, \n   \"B\" -> 12, \"\\[Theta]\" -> 90.000000000000", 8084="\"\\[Zeta]\" -> 0.027897403691, \"\\[Tau]1\" -> 0.014639690770, \n   \"\\[Tau]S\" -> 0.004105291179, \"\\[Tau]N\" -> 0.000006999171, \n   \"\\[Tau]C\" -> 0.007414449545, \"\\[Kappa]0\" -> 0.000000059701, \n   \"mm1\" -> 0.000000000000, \"mm2\" -> 0.000000000000, \n   \"mm3\" -> 0.000000000000, \"T\" -> 6.000000000000, \n   \"B\" -> 12, \"\\[Theta]\" -> 90.000000000000"}
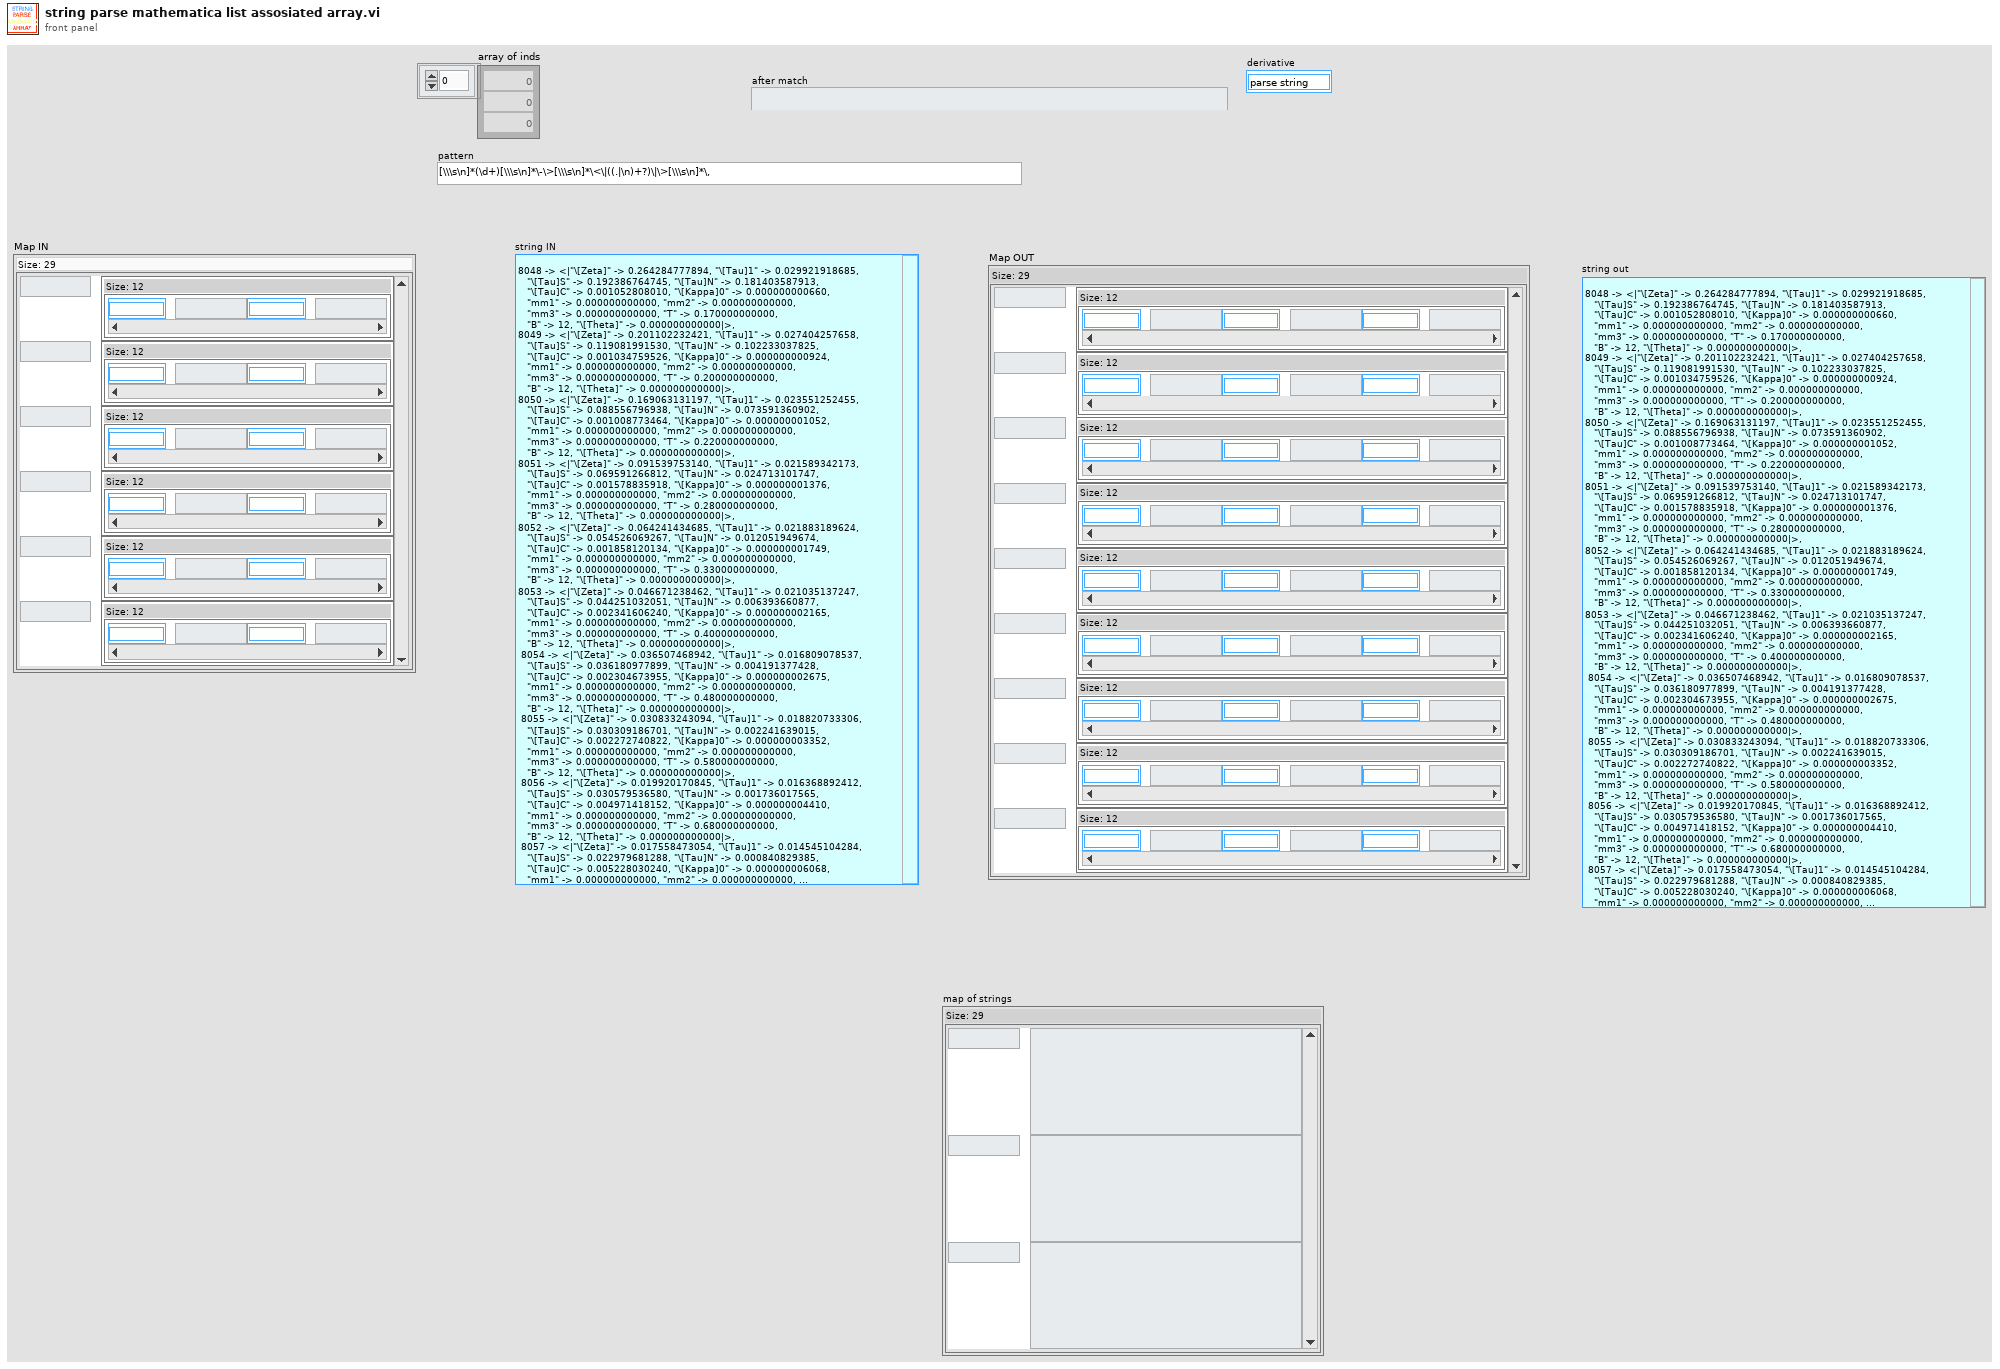
[diagram p1: front panel]
types:
  T1 = typedef "3-lorentzian-parameters.ctl" = enum16{"ζ", "τ1", "τS", "τN", "τC", "κ0", "m1", "m2", "m3", "T (K)", "B (T)", "θ (deg)", "side (S|R)", "change (B|T)"}
  T2 = typedef "3-lorentzian-heat-response action.ctl" = enum16{"calc R", "create string", "calc m1m2m3", "dζ", "dT1", "dτS", "dτN", "dτC", "d-all", "dκ0", "T(K)", "m1", "m2", "m3", "parse string", "θ (deg)", "B (T)", "onlygrads", "newton", "create emty string"}
  T3 = typedef "mathematica string map action.ctl" = enum16{"create string", "calc m1m2m3", "parse string"}
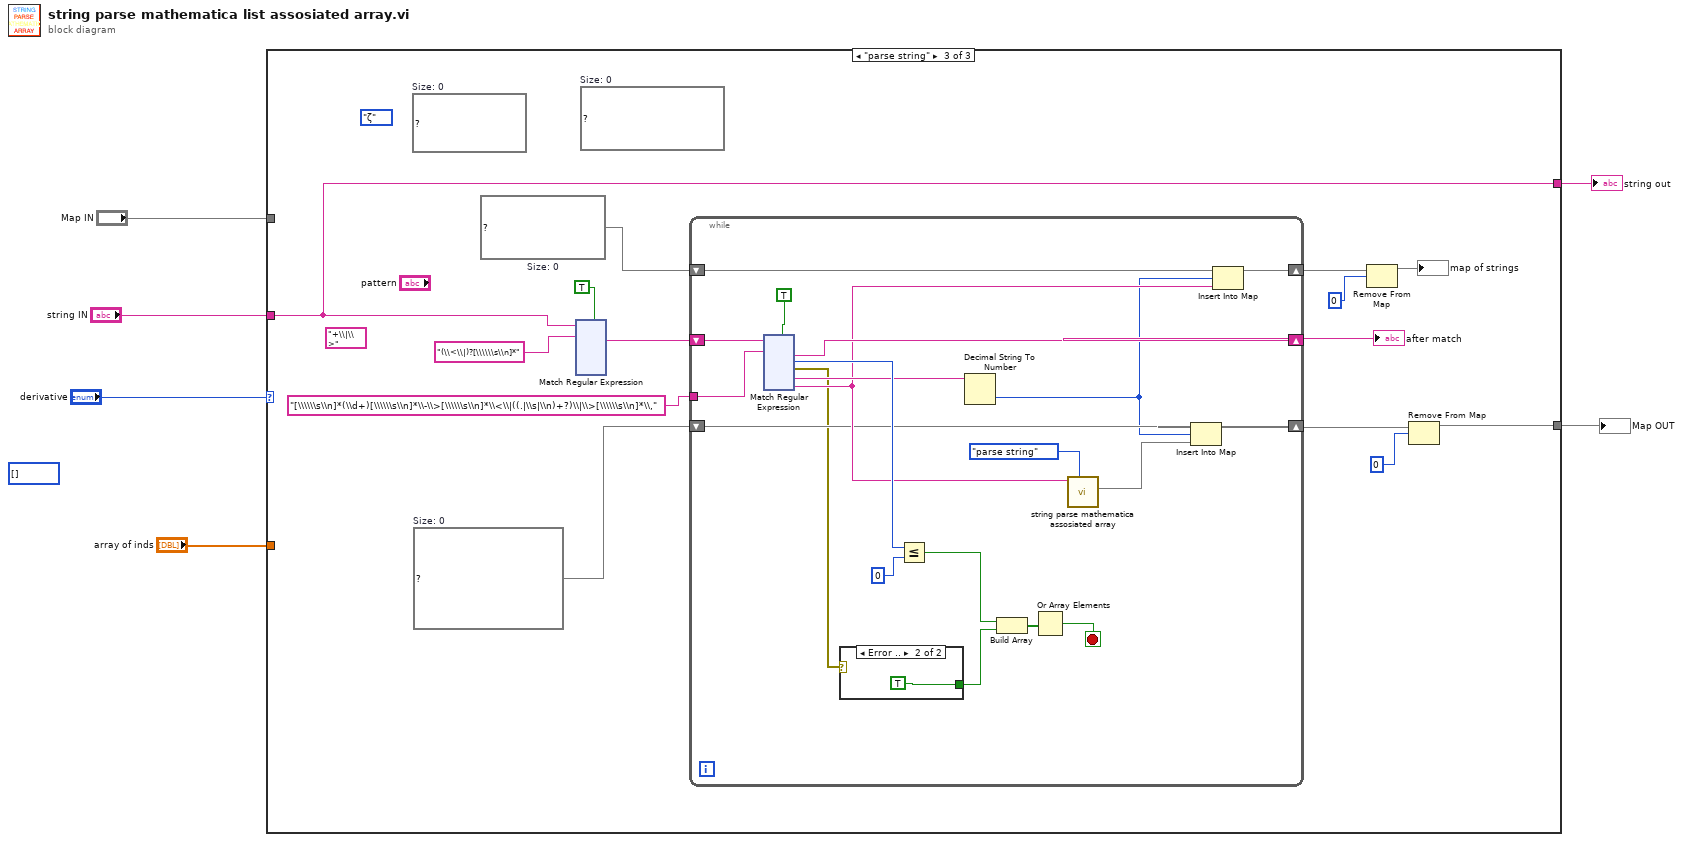
[diagram p0: block diagram]
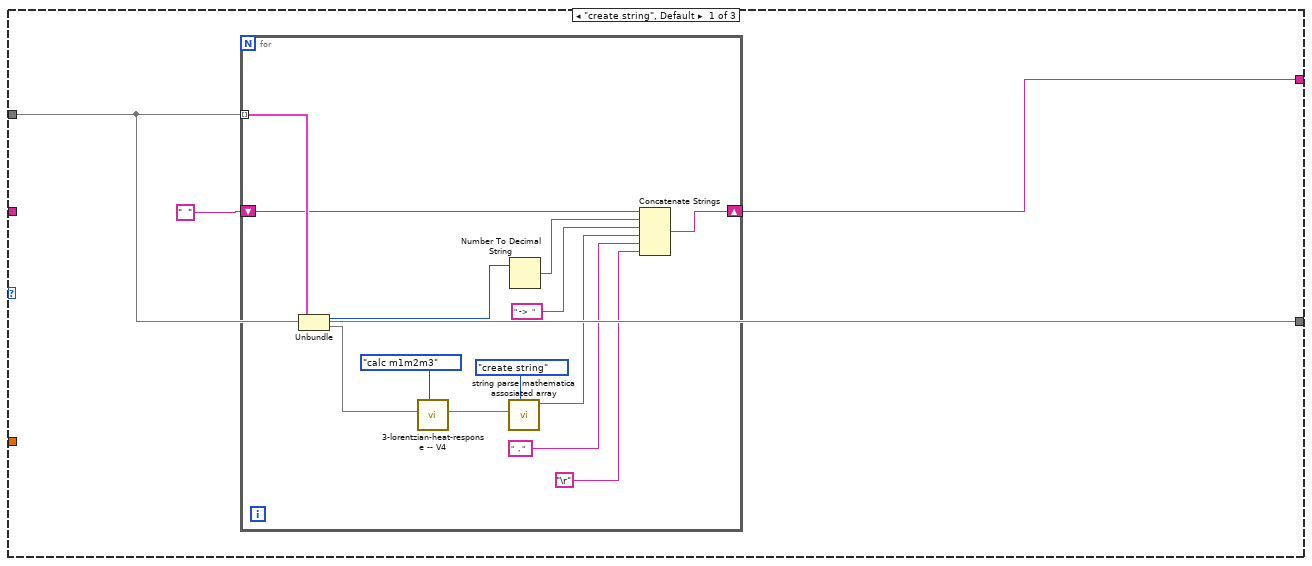
[diagram p2: hidden frame]
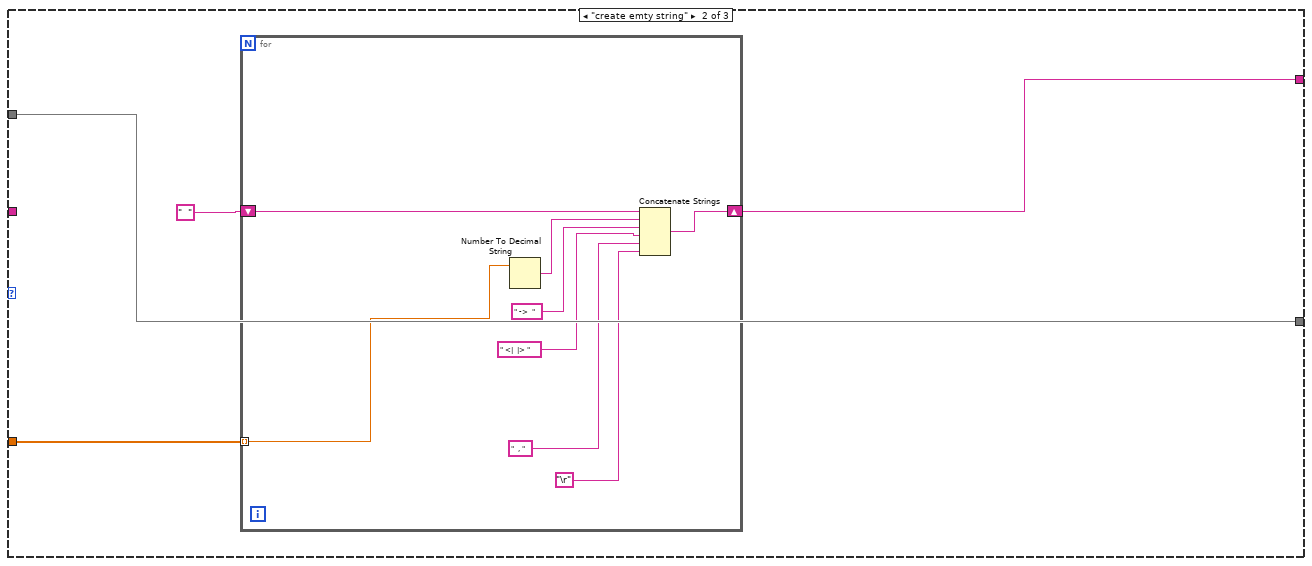
[diagram p3: hidden frame]
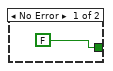
[diagram p4: hidden frame]
diagram:
  (unwired) i32[] []
  n1 = case shown="\"parse string\"" "derivative" {
    tunnel: "string IN" -> [_ _ w37]
    tunnel: [w7 w24 w38] -> w5
    tunnel: "Map IN" -> [w7 w24 _]
    tunnel: [w9 w26 w37] -> w2
    tunnel: "array of inds" -> [_ w23 _]
    frame "create string", Default {
      n2 = for {
        tunnel: w7 -> [w22] mode=indexing
        shift-right: [w14] -> w9
        shift-left: "  " ("all string") -> [w15]
        n3 = Unbundle(w22) -> ("index"=w21:i32, "Map"=w12:map{T1, dbl})
        n4 = call "3-lorentzian-heat-response -- V4.vi"("action"=3-lorentzian-heat-response_action."calc m1m2m3", "Map IN"=w12) -> ("Map OUT"=w10:map{T1, dbl})  [unwired: 7 in, 2 out]
        n5 = call "string parse mathematica assosiated array.vi"("derivative"=mathematica_string_map_action."create string", "Map IN"=w10) -> ("String OUT"=w18:string)  [unwired: 8 in, 1 out]
        n6 = Number To Decimal String(number=w21) -> (decimal integer string=w20:string)  [unwired: 1 in]
        n7 = Concatenate Strings(w15, w20, " ->  " ("all string"), w18, "  , " ("all string"), "\r") -> (w14:string)
      }
    }
    frame "create emty string" {
      n8 = for {
        shift-right: [w30] -> w26
        shift-left: "  " ("all string") -> [w31]
        tunnel: w23 -> [w28] mode=indexing
        n9 = Number To Decimal String(number=w28) -> (decimal integer string=w34:string)  [unwired: 1 in]
        n10 = Concatenate Strings(w31, w34, " ->  " ("all string"), " <|  |> " ("all string"), "  , " ("all string"), "\r") -> (w30:string)
      }
    }
    frame "parse string" {
      (unwired) 3-lorentzian-parameters."ζ" ("X selector")
      w44 = map{i32, map{T1, dbl}} {}  # Size: 0
      w46 = map{i32, string} {}  # Size: 0
      (unwired) "+\\|\\>" ("format string")
      (unwired) map{T1, dbl} {}  # Size: 0
      (unwired) map{T1, string} {}  # Size: 0
      n11 = xnode "Match Regular Expression"("input string"=w37, "regular expression"="(\\<\\|)?[\\\\\\s\\n]*" ("format string"), "multiline? (F)"=TRUE) -> ("after match"=w47:string)  [unwired: 3 in, 6 out]
      n12 = while {
        shift-right: [w65] -> w45
        shift-left: w47 -> [w68]
        tunnel: "[\\\\\\s\\n]*(\\d+)[\\\\\\s\\n]*\\-\\>[\\\\\\s\\n]*\\<\\|((.|\\s|\\n)+?)\\|\\>[\\\\\\s\\n]*\\," ("pattern") -> [w64]
        shift-right: [w61] -> w43
        shift-left: w46 -> [w63]
        shift-right: [w55] -> w39
        shift-left: w44 -> [w58]
        stop <- w51 stop-if-true
        n13 = xnode "Match Regular Expression"("input string"=w68, "regular expression"=w64, "multiline? (F)"=TRUE) -> ("after match"=w65:string, "offset past match"=w67:i32, "error out"=w52:errorcluster, "submatch 1"=w62:string, "submatch 2"=w59:string)  [unwired: 3 in, 2 out]
        n14 = case shown="Error .." w52 {
          tunnel: [FALSE TRUE] -> w49
          frame No Error {
          }
          frame Error {
          }
        }
        n15 = Less Or Equal?(x=w67, y=0) -> (x <= y?=w53:bool)
        n16 = Decimal String To Number(string=w62) -> (number=w57:i32)  [unwired: 2 in, 1 out]
        n17 = Build Array(w53, w49) -> (w50:bool[])
        n18 = Or Array Elements(Boolean array=w50) -> (logical OR=w51:bool)
        n19 = call "string parse mathematica assosiated array.vi"("derivative"=mathematica_string_map_action."parse string", "String in"=w59) -> ("Map OUT"=w56:map{T1, dbl})  [unwired: 8 in, 1 out]
        n20 = Insert Into Map(map in=w58, key=w57, value=w56) -> (map out=w55:map{i32, map{T1, dbl}})  [unwired: 2 out]
        n21 = Insert Into Map(map in=w63, key=w57, value=w59) -> (map out=w61:map{i32, string})  [unwired: 2 out]
      }
      "after match" <- w45
      n22 = Remove From Map(10:0 ("key"), 11:w43) -> (3:→"map of strings":map{i32, string})  [unwired: 2 out]
      n23 = Remove From Map(10:0 ("key"), 11:w39) -> (3:w38:map{i32, map{T1, dbl}})  [unwired: 2 out]
    }
  }
  "Map OUT" <- w5
  "string out" <- w2
